vi "Build Database Path.vi"(6 "DB Type":u16, 8 "Error In":errorcluster, 9 "Selected Library Names":string[](array[string]), 11 "Folder containing database files":path=path "C:/Ehsan Temp Folder/TFS/LV/Data Logging with LabVIEW/SV names.csv") -> (0 "Error Out":errorcluster, 1 "Database not available for at least one?":bool, 2 "Database Availability for selected libraries":bool[](array[boolean]), 3 "Database path array for selected libraries":path[](array[path]), 4 "More than one database?":bool[](array[boolean]))   [LabVIEW 2014]
doc: "<B>Copyright</B>: (c) MHWirth 2015. All rights are reserved."
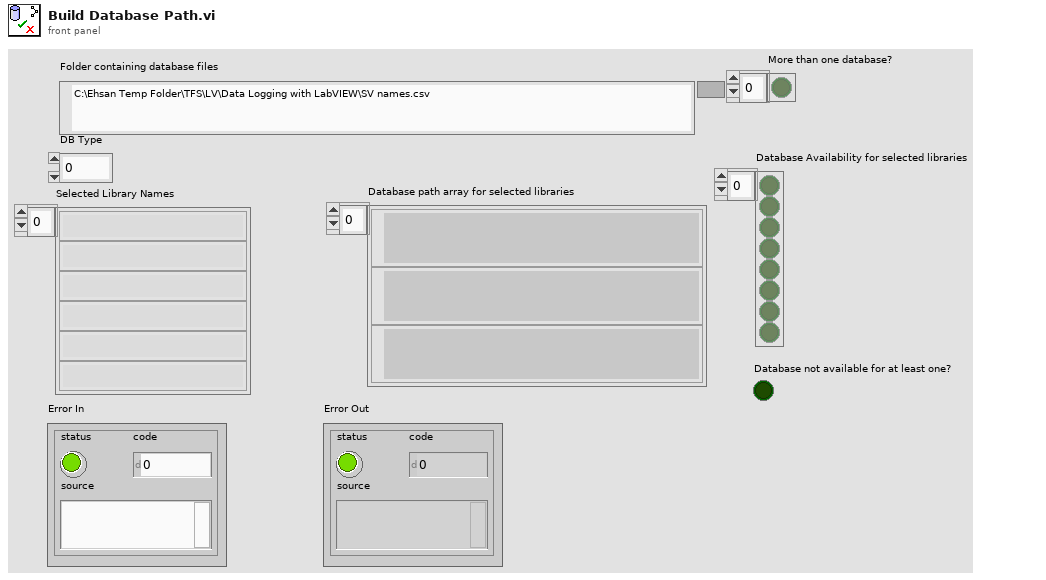
[diagram p1: front panel]
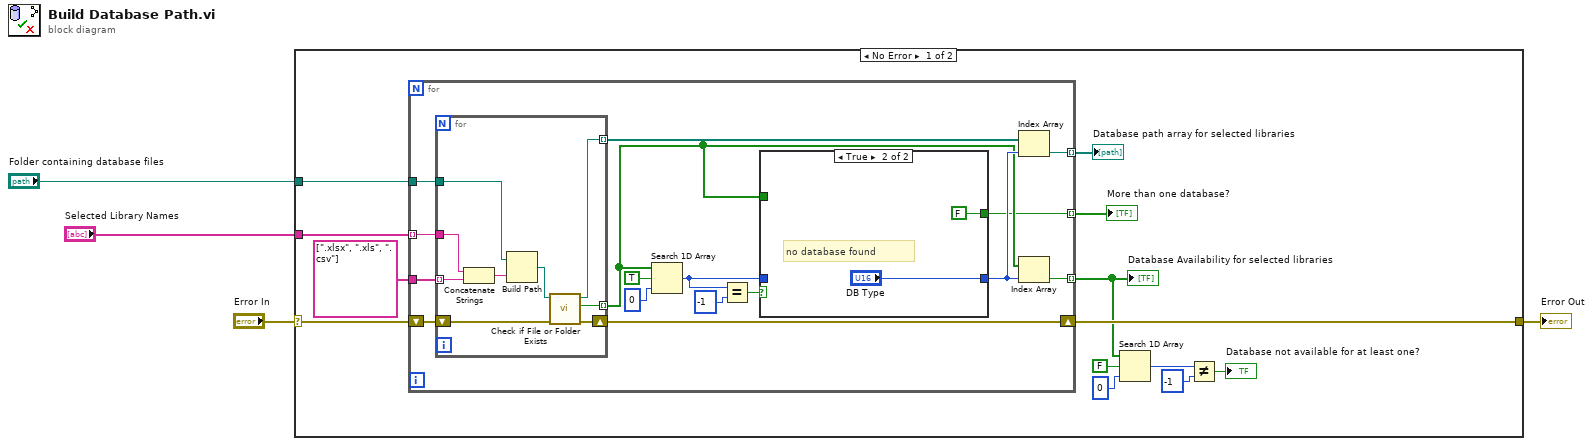
[diagram p0: block diagram]
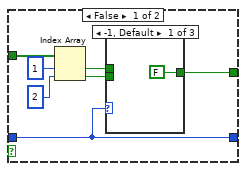
[diagram p2: hidden frame]
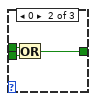
[diagram p3: hidden frame]
diagram:
  n1 = case shown="No Error" "Error In" {
    selector: "Error In" -> [w15 w57]
    tunnel: "Folder containing database files" -> [w16 _]
    tunnel: "Selected Library Names" -> [w17 _]
    tunnel: [w9 w57] -> w1
    frame No Error {
      n2 = for {
        tunnel: w17 -> [w33] mode=indexing
        tunnel: w16 -> [w32]
        shift-right: [w30] -> w9
        shift-left: w15 -> [w31]
        tunnel: string[] [".xlsx", ".xls", ".csv"] -> [w29]
        tunnel: [w24] -> w7 mode=indexing
        tunnel: [w23] -> w5 mode=indexing
        tunnel: [w18] -> w6 mode=indexing
        n3 = for {
          tunnel: w33 -> [w56]
          tunnel: [w52] -> w19 mode=indexing
          shift-right: [w50] -> w30
          shift-left: w31 -> [w51]
          tunnel: w32 -> [w54]
          tunnel: [w49] -> w25 mode=indexing
          tunnel: w29 -> [w48] mode=indexing
          n4 = Concatenate Strings(w56, w48) -> (w55:string)
          n5 = Build Path(base path=w54, name or relative path=w55) -> (appended path=w53:path)
          n6 = call <vilib>:"Check if File or Folder Exists.vi"("error in (no error)"=w51, "path"=w53) -> ("error out"=w50:errorcluster, "file or folder exists?"=w52:bool, "dup path"=w49:path)  [unwired: 7 in]
        }
        n7 = Search 1D Array(1D array=w19, element=TRUE, start index (0)=0) -> (index of element=w21:i32)
        n8 = Equal?(x=w21, y=-1) -> (x = y?=w22:bool)
        n9 = case shown="True" w22 {
          tunnel: w21 -> [w40 _]
          tunnel: [w40 "DB Type"] -> w20
          tunnel: w19 -> [w39 _]
          tunnel: [w34 FALSE ("file or folder exists?")] -> w18
          frame False {
            n10 = Index Array(array=w39, index #1=1 ("index"), index #2=2 ("index")) -> (element #1=w36:bool, element #2=w35:bool)
            n11 = case shown="-1, Default" w40 {
              tunnel: w36 -> [_ w44 _]
              tunnel: w35 -> [_ w43 w45]
              tunnel: [FALSE ("file or folder exists?") w42 w45] -> w34
              frame -1, Default {
              }
              frame 0 {
                n12 = Or(x=w44, y=w43) -> (x .or. y?=w42:bool)
              }
              frame 1 {
              }
            }
          }
          frame True {
            # "no database found"
          }
        }
        n13 = Index Array(array=w25, index=w20) -> (element=w24:path)
        n14 = Index Array(array=w19, index=w20) -> (element=w23:bool)
      }
      "Database path array for selected libraries" <- w7
      "Database Availability for selected libraries" <- w5
      "More than one database?" <- w6
      n15 = Search 1D Array(1D array=w5, element=FALSE, start index (0)=0) -> (index of element=w12:i32)
      n16 = Not Equal?(x=w12, y=-1) -> (x != y?=→"Database not available for at least one?":bool)
    }
    frame Error {
    }
  }
  "Error Out" <- w1
